vi "CustomMask.vi"(2 "error in (no error)":errorcluster, 3 "Custom Mask":u32[](array[numeric]), 4 "VISA resource name":refnum<visa-resource-name>) -> (0 "error out":errorcluster, 1 "VISA resource name out":refnum<visa-resource-name>)   [LabVIEW 2012]
doc: "Sends commands to the cyberglove to mask a custom array of sensors."
panel:
  out "string":string
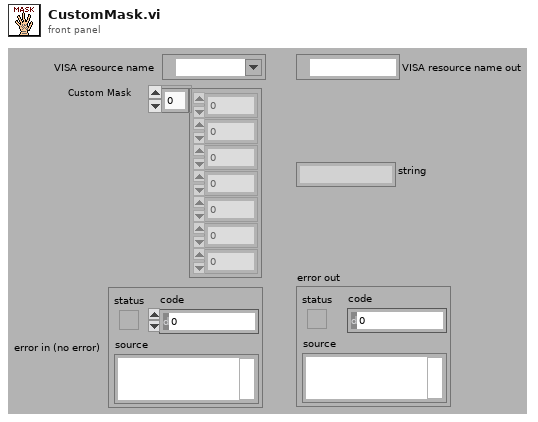
[diagram p1: front panel]
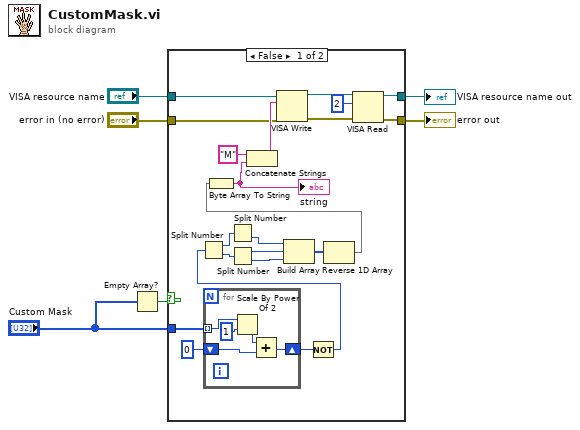
[diagram p0: block diagram]
diagram:
  n1 = Empty Array?(array="Custom Mask") -> (empty?=w1:bool)
  n2 = case shown="False" w1 {
    tunnel: "VISA resource name" -> [w20 w34]
    tunnel: "error in (no error)" -> [w19 w33]
    tunnel: [w14 w34] -> w4
    tunnel: [w13 w33] -> w5
    tunnel: "Custom Mask" -> [w27 _]
    frame False {
      n3 = for {
        tunnel: w27 -> [w30] mode=indexing
        shift-right: [w31] -> w18
        shift-left: u32 0 ("y") -> [w32]
        n4 = Scale By Power Of 2(n=w30, x=u32 1) -> (x*2^n=w28:u32)
        n5 = Add(x=w28, y=w32) -> (x+y=w31:u32)
      }
      n6 = Not(x=w18) -> (.not. x?=w17:u32)
      n7 = Split Number(x=w17) -> (hi(x)=w25:u16, lo(x)=w24:u16)
      n8 = Split Number(x=w25) -> (lo(x)=w11:u8)  [unwired: 1 out]
      n9 = Split Number(x=w24) -> (hi(x)=w10:u8, lo(x)=w9:u8)
      n10 = Build Array(w11, w10, w9) -> (w8:u8[])
      n11 = Reverse 1D Array(array=w8) -> (reversed array=w7:u8[])
      n12 = Byte Array To String(unsigned byte array=w7) -> (string=w22:string)
      "string" <- w22
      n13 = Concatenate Strings("M" ("string"), w22) -> (w21:string)
      n14 = VISA Write(VISA resource name=w20, write buffer=w21, error in (no error)=w19) -> (VISA resource name out=w16:refnum<visa-resource-name>, error out=w15:errorcluster)  [unwired: 1 out]
      n15 = VISA Read(VISA resource name=w16, byte count=u32 2, error in (no error)=w15) -> (VISA resource name out=w14:refnum<visa-resource-name>, error out=w13:errorcluster)  [unwired: 2 out]
    }
    frame True {
    }
  }
  "error out" <- w5
  "VISA resource name out" <- w4
